vi "data.vi"() -> ()   [LabVIEW 2019]
uses:
  <vilib>/Platform/TimedLoop/XDataNode/timing_clust.ctl
  <vilib>/Platform/TimedLoop/XDataNode/nitl_modes.ctl
  <vilib>/Platform/TimedLoop/XDataNode/wakeup.ctl
  <vilib>/Analysis/baseanly.llb/Mean (DBL).vi
  <vilib>/platform/TimedLoop/XDataNode/XDataNode.xnode
  <vilib>/Platform/TimedLoop/XDataNode/XDNodeRunTimeDep.lvlib
  <vilib>/Analysis/NI_AALBase.lvlib
panel:
  out "mean":dbl format="%0.2f"
  out "min value":dbl
  out "max value":dbl
  in  "Ready":bool
  out "Waveform Graph":dynamicdata(graph)
  out "Live Signal":dbl(graph)
  out "Data":dbl
  in  "Unit Change":bool
  out "Current data point":dbl
  in  "stop":bool
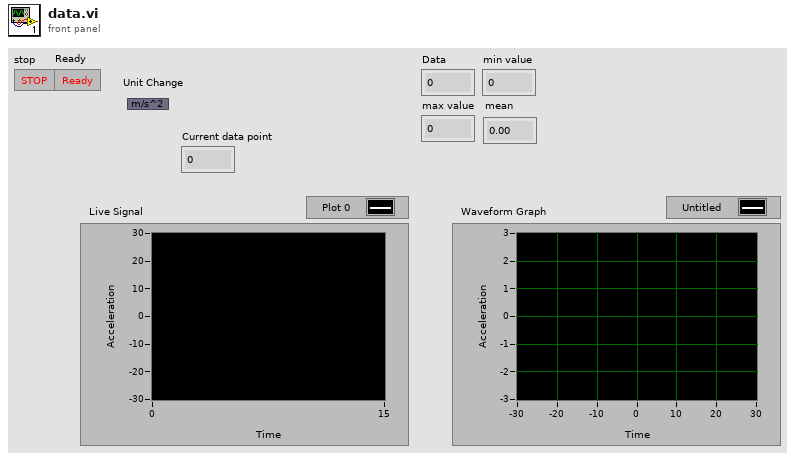
[diagram p1: front panel]
types:
  T1 = typedef "XDNodeRunTimeDep.lvlib/timing_clust.ctl" = cluster{"Expected End [f-1]":u64, "Actual End [f-1]":u64, "Finished Late? [f-1]":bool, "Expected End [i-1]":u64, "Actual End [i-1]":u64, "Finished Late? [i-1]":bool, "Expected Start [i]":u64, "Actual Start [i]":u64, "Expected Start [f]":u64, "Actual Start [f]":u64, "Source Name":string, "Structure Name":string, "Period":i64, "Deadline":i64, "Offset":i64, "Start":i64, "Priority":i32, "Timeout":i32, "Mode":T2, "Wakeup Reason":T3, "Error":errorcluster, "Source Type":string, "Secondary Source Type":string, "Global End Time":u64, "Global Start Time":u64, "Frame Duration":u64, "Iteration Duration":u64, "Assigned CPU":i32, "I/O Scan Engine Mode":u32}
  T2 = typedef "XDNodeRunTimeDep.lvlib/nitl_modes.ctl" = enum32{"No Change", "Process missed periods, maintain original phase", "Discard missed periods, maintain original phase", "Process missed periods, ignore original phase", "Discard missed periods, ignore original phase"}
  T3 = typedef "XDNodeRunTimeDep.lvlib/wakeup.ctl" = enum32{"Normal", "Aborted", "Asynchronous wakeup", "Timing source error", "Timed loop error", "Timeout"}
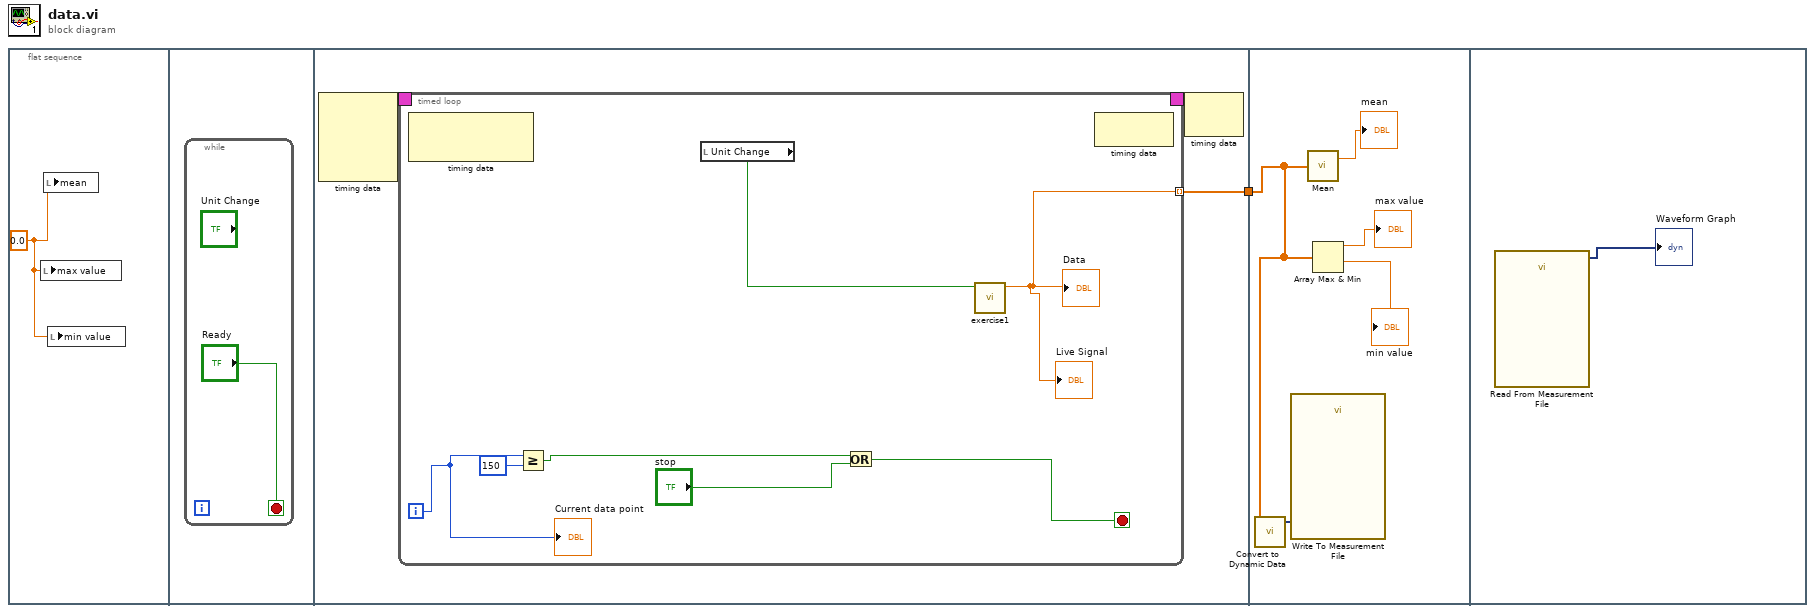
[diagram p0: block diagram]
diagram:
  n1 = flat-sequence {
    tunnel: [w4] -> w1
    tunnel: w1 -> [w19]
    frame #0 {
      w2 = 0.0 ("mean")
      n2 = local write "max value"(w2) -> ()
      n3 = local write "mean"(w2) -> ()
      n4 = local write "min value"(w2) -> ()
    }
    frame #1 {
      n5 = while {
        stop <- "Ready" stop-if-true
      }
    }
    frame #2 {
      n6 = node-c288() -> (w6:T1)  [unwired: 4 in]
      n7 = timed-loop {
        timing: w6 -> [_]
        timing-out: [_] -> w5
        tunnel: [w7] -> w4 mode=indexing
        i -> [w9]
        stop <- w10 stop-if-true
        n8 = node-c288() -> ()  [unwired: 1 in, 2 out]
        n9 = Greater Or Equal?(x=w9, y=150) -> (x >= y?=w11:bool)
        n10 = local read "Unit Change"() -> (w8:bool)
        n11 = Or(x=w11, y="stop") -> (x .or. y?=w10:bool)
        n12 = call "exercise1.vi"("Acceleration in m/s^2 or g"=w8) -> ("Data"=w7:dbl)  [unwired: 10 in]
        "Data" <- w7
        "Live Signal" <- w7
        n13 = node-c288() -> ()  [unwired: 1 in, 1 out]
        "Current data point" <- w9
      }
      n14 = node-c288(w5) -> ()  [unwired: 1 out]
    }
    frame #3 {
      n15 = call "Convert to Dynamic Data"("Array"=w19) -> ("Dynamic Data Type"=w18:dynamicdata)  [unwired: 3 in]
      n16 = call "Write To Measurement File"("Signals"=w18) -> ()  [unwired: 16 in, 3 out]
      n17 = call-poly <vilib>:"Mean.vi"("X"=w19) -> ("mean"=→"mean":dbl)  [unwired: 1 out]
      n18 = Array Max & Min(array=w19) -> (max value=→"max value":dbl, min value=→"min value":dbl)  [unwired: 2 out]
    }
    frame #4 {
      n19 = call "Read From Measurement File"() -> ("Signals"=→"Waveform Graph":dynamicdata)  [unwired: 6 in, 5 out]
    }
  }
